vi "Initialize Instrument.vi"(8 "error in (no error)":errorcluster, 10 "Instr Resource Str":string, 11 "Tek 2k.lvclass in":refnum<class "Tek 2k Scope.lvclass">) -> (0 "error out":errorcluster, 3 "Tek 2k.lvclass out":refnum<class "Tek 2k Scope.lvclass">)   [LabVIEW 2010, in "Tek 2k Scope.lvclass"]
uses:
  Tek 2k Scope.lvclass
  Tek 2k Scope.lvclass/Tek 2k Scope.ctl
  <instrlib>/Tektronix TDS 200 1000 2000 Series/Tektronix TDS 200 1000 2000 Series.lvlib
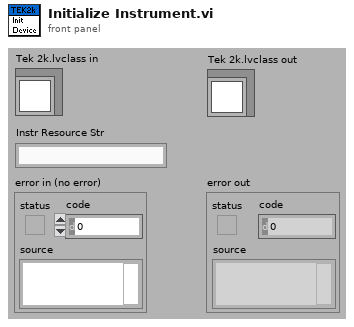
[diagram p1: front panel]
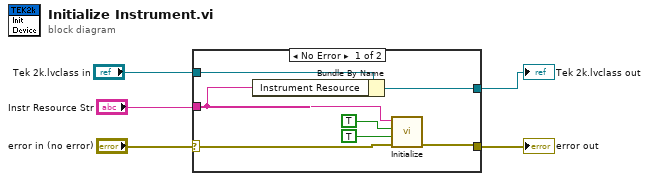
[diagram p0: block diagram]
diagram:
  n1 = case shown="No Error" "error in (no error)" {
    selector: "error in (no error)" -> [w10 w14]
    tunnel: [w9 w14] -> w5
    tunnel: "Instr Resource Str" -> [w8 _]
    tunnel: "Tek 2k.lvclass in" -> [w7 w13]
    tunnel: [w6 w13] -> w1
    frame No Error {
      n2 = Bundle By Name(cluster=w7, "Instrument Resource"=w8) -> (w6:refnum<class "Tek 2k Scope.lvclass">)
      n3 = call <instrlib>:"Initialize.vi"("error in (no error)"=w10, "Reset? (T: Yes)"=TRUE, "ID Query? (T: Yes)"=TRUE, "VISA resource name"=w8) -> ("error out"=w9:errorcluster)  [unwired: 1 in, 6 out]
    }
    frame Error {
    }
  }
  "error out" <- w5
  "Tek 2k.lvclass out" <- w1
